vi "Check Refnum Class.vi"(8 "error in (no error)":errorcluster, 11 "Text field in":refnum<class "Text field.lvclass">) -> (0 "error out":errorcluster, 3 "Text field out":refnum<class "Text field.lvclass">)   [LabVIEW 2020, in "Text field.lvclass"]
uses:
  Text field.lvclass
  C:/Users/User/Desktop/Raman Program/Database OOP/source/Field/Field.lvclass
  Field.lvclass/Field.ctl
  Field.lvclass
panel:
  # "For override: make sure that the wired control refnum class matches the field child class"
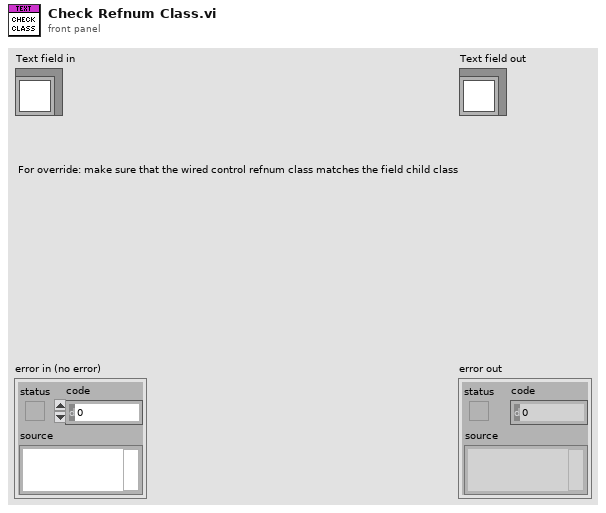
[diagram p1: front panel]
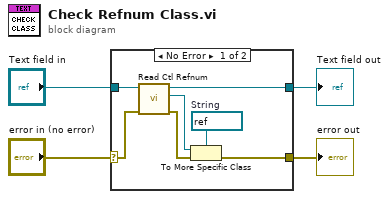
[diagram p0: block diagram]
diagram:
  n1 = case shown="No Error" "error in (no error)" {
    selector: "error in (no error)" -> [w8 w12]
    tunnel: "Text field in" -> [w11 w13]
    tunnel: [w5 w13] -> w3
    tunnel: [w6 w12] -> w1
    frame No Error {
      w9 = refnum<vi> refnum  # String
      n2 = call "Read Ctl Refnum.vi"("error in (no error)"=w8, "Field in"=w11) -> ("error out"=w7:errorcluster, "Ctl Refnum"=w10:refnum<vi>, "Field out"=w5:refnum<class "Text field.lvclass">)  [unwired: 7 in]
      n3 = To More Specific Class(target class=w9, reference=w10, error in=w7) -> (error out=w6:errorcluster)  [unwired: 1 out]
    }
    frame Error {
    }
  }
  "error out" <- w1
  "Text field out" <- w3
